vi "Teleop.vi"(10 "Match Info":T1={"Autonomous Elapsed Seconds"=0.0, "TeleOp Elapsed Seconds"=0.0, "Disabled Elapsed Seconds"=0.0, "Visited Autonomous"=FALSE, "Visited TeleOp"=FALSE, "Visited Disabled"=FALSE, "Autonomous Settings"={"Autonomous Style"=enum."Independent", "VI Refnum"=refnum}}, 11 "Call Context":T2=enum."Stop") -> ()   [LabVIEW 2019]
doc: "This VI is called for each enabled TeleOp packet received from the DS. It is typically used to read from joysticks and other inputs and update I/O or setpoints for timed control loops. It should complete and return within 20 milliseconds or risk missing DS packets."
uses:
  <vilib>/Rock Robotics/WPI/DriverStation/WPI_DriverStationDerivedRobotMode.ctl
  <vilib>/Rock Robotics/WPI/DriverStation/WPI_DriverStationMatch Info.ctl
  Typedef/XBox Axis.ctl
  Typedef/XBox Buttons.ctl
  Typedef/XBox POV.ctl
  <vilib>/Rock Robotics/WPI/Utilities/WPI_GetSetVariantRefNum.vi
  <vilib>/Rock Robotics/Network Tables/NT Write Boolean Array.vi
  <vilib>/Rock Robotics/Network Tables/NT Write Numeric Array.vi
panel:
  in  "Winch Speed":dbl=-0.6
  in  "Climb Up Speed":dbl
  in  "Climb Down Speed":dbl
  in  "Queso Arc Sensitivty":dbl=0.5
  in  "QuickTurn Sensitivty":dbl=0.7
  in  "Throttle Sensitivity":dbl=0.5
  in  "max queso power (1)":dbl=1.0
  in  "Trigger Threshold":dbl=0.5 format="%#_13g"
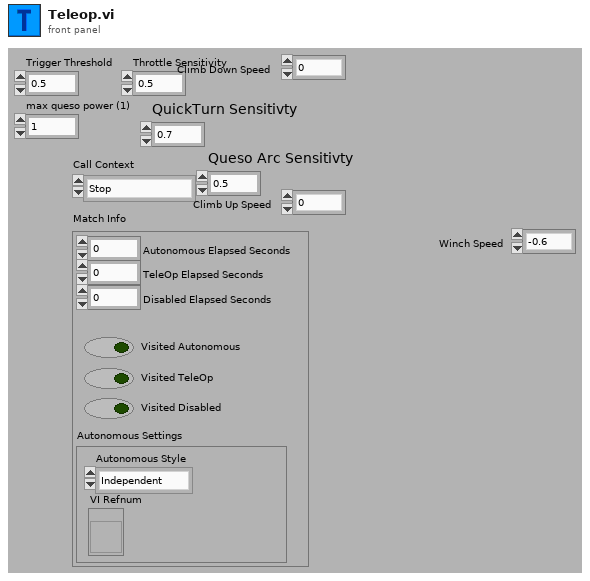
[diagram p1: front panel]
types:
  T1 = typedef "WPI_DriverStationMatch Info.ctl" = cluster{"Autonomous Elapsed Seconds":dbl, "TeleOp Elapsed Seconds":dbl, "Disabled Elapsed Seconds":dbl, "Visited Autonomous":bool, "Visited TeleOp":bool, "Visited Disabled":bool, "Autonomous Settings":cluster{"Autonomous Style":enum16{"Iterative", "Independent"}, "VI Refnum":refnum<vi>}}
  T2 = typedef "WPI_DriverStationDerivedRobotMode.ctl" = enum16{"Init", "Execute", "Stop"}
  T3 = typedef "XBox Buttons.ctl" = enum16{"A", "B", "X", "Y", "Left Bumper", "Right Bumper", "Back", "Start", "Left Joystick", "Right Joystick"}
  T4 = typedef "XBox Axis.ctl" = enum16{"Left X", "Left Y", "Left Trigger", "Right Trigger", "Right X", "Right Y"}
  T5 = typedef "XBox POV.ctl" = enum16{"Center", "Top", "Top Right", "Center Right", "Bottom Right", "Bottom", "Bottom Left", "Center Left", "Top Left"}
  T6 = typedef "WPI_JoystickDevRef.ctl" = cluster{"Device":T7}
  T7 = typedef "WPI_JoystickDeviceEnum.ctl" = enum16{"USB 0", "USB 1", "USB 2", "USB 3", "USB 4", "USB 5"}
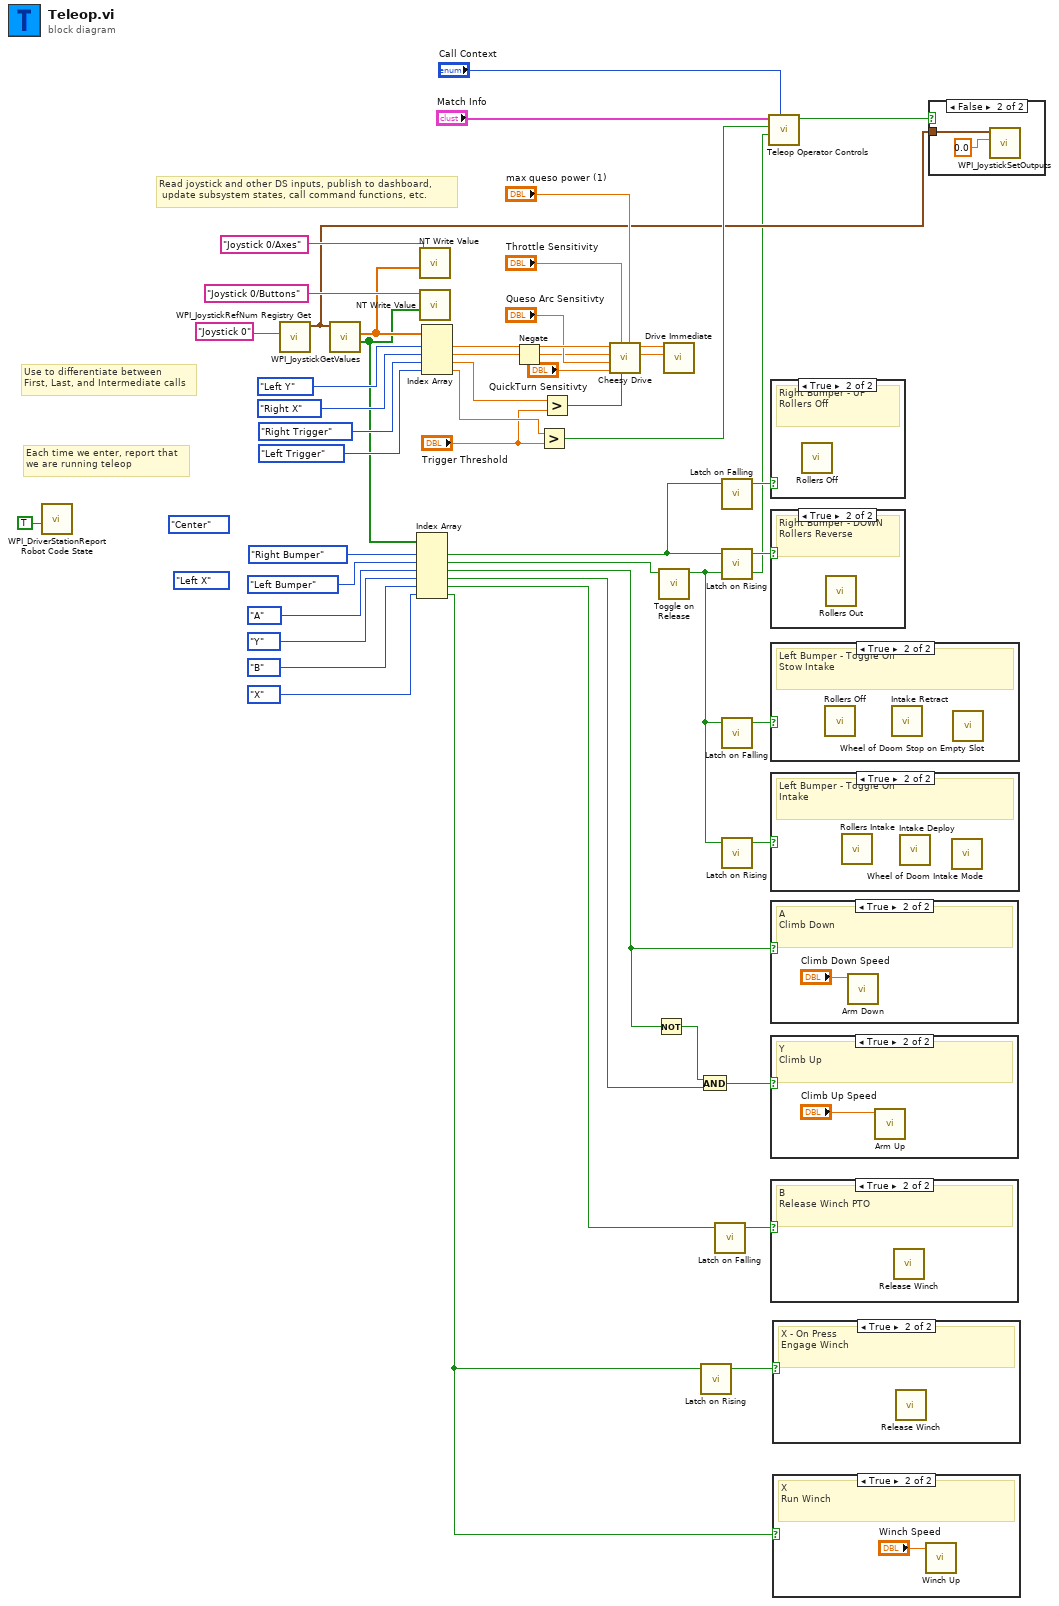
[diagram p0: block diagram]
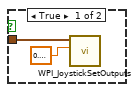
[diagram p7: hidden frame]
diagram:
  (unwired) XBox_Axis."Left X" ("Enum 3")
  (unwired) XBox_POV."Center" ("Enum")
  # "Read joystick and other DS inputs, publish to dashboard,\n update subsystem states, call command functions, etc."
  # "Each time we enter, report that\nwe are running teleop"
  # "Use to differentiate between\nFirst, Last, and Intermediate calls"
  n1 = call <vilib>:"WPI_DriverStationReport Robot Code State.vi"("TeleOp"=TRUE ("Autonomous")) -> ()  [unwired: 10 in, 1 out]
  n2 = call <vilib>:"WPI_JoystickRefNum Registry Get.vi"("refnum name"="Joystick 0") -> ("JoystickDevRef"=w15:T6)  [unwired: 1 in, 9 out]
  n3 = call <vilib>:"WPI_JoystickGetValues.vi"("JoystickDevRef"=w15) -> ("Buttons"=w35:bool[], "Axes"=w46:dbl[])  [unwired: 6 in, 3 out]
  n4 = Index Array(array=w35, index #1=XBox_Buttons."Right Bumper" ("Enum 2"), index #2=XBox_Buttons."Left Bumper" ("Enum 2"), index #3=XBox_Buttons."A" ("Enum 2"), index #4=XBox_Buttons."Y" ("Enum 2"), index #5=XBox_Buttons."B" ("Enum 2"), index #6=XBox_Buttons."X" ("Enum 2")) -> (element #1=w30:bool, element #2=w26:bool, element #3=w8:bool, element #4=w6:bool, element #5=w3:bool, element #6=w1:bool)
  n5 = call-poly <vilib>:"NT Write Value.vi"("Numeric Array"=w46, "Name"="Joystick 0/Axes") -> ()  [unwired: 9 in, 1 out]
  n6 = call-poly <vilib>:"NT Write Value.vi"("Boolean Array"=w35, "Name"="Joystick 0/Buttons") -> ()  [unwired: 9 in, 1 out]
  n7 = Index Array(array=w46, index #1=XBox_Axis."Left Y" ("Enum"), index #2=XBox_Axis."Right X" ("Enum"), index #3=XBox_Axis."Right Trigger" ("Enum"), index #4=XBox_Axis."Left Trigger" ("Enum")) -> (element #1=w39:dbl, element #2=w38:dbl, element #3=w34:dbl, element #4=w25:dbl)
  n8 = Negate(x=w38) -> (-x=w18:dbl)
  n9 = Greater?(x=w25, y="Trigger Threshold") -> (0:w23:bool)
  n10 = Greater?(x=w34, y="Trigger Threshold") -> (0:w33:bool)
  n11 = call <vilib>:"Cheesy Drive.vi"("max queso power (1)"="max queso power (1)", "Quickturn"=w33, "Throttle Sensitivity"="Throttle Sensitivity", "QuickTurn Sensitivty"="QuickTurn Sensitivty", "Queso Arc Sensitivty"="Queso Arc Sensitivty", "Wheel"=w18, "Throttle"=w39) -> ("Right PWM"=w36:dbl, "Left PWM"=w37:dbl)  [unwired: 3 in]
  n12 = Not(x=w8) -> (.not. x?=w7:bool)
  n13 = call <vilib>:"Toggle on Release.vi"("Boolean"=w26) -> ("toggle on release"=w14:bool)  [unwired: 10 in]
  n14 = call "Drive Immediate.vi"("Right Setpoint"=w36, "Left Setpoint"=w37) -> ()  [unwired: 9 in, 1 out]
  n15 = And(x=w7, y=w6) -> (x .and. y?=w5:bool)
  n16 = call <vilib>:"Latch on Rising.vi"("Boolean in"=w1) -> ("Boolean out"=w2:bool)  [unwired: 4 in]
  n17 = call <vilib>:"Latch on Falling.vi"("Boolean in"=w3) -> ("Boolean out"=w4:bool)  [unwired: 4 in]
  n18 = call <vilib>:"Latch on Falling.vi"("Boolean in"=w30) -> ("Boolean out"=w31:bool)  [unwired: 4 in]
  n19 = call <vilib>:"Latch on Rising.vi"("Boolean in"=w30) -> ("Boolean out"=w29:bool)  [unwired: 4 in]
  n20 = call <vilib>:"Latch on Falling.vi"("Boolean in"=w14) -> ("Boolean out"=w27:bool)  [unwired: 4 in]
  n21 = call <vilib>:"Latch on Rising.vi"("Boolean in"=w14) -> ("Boolean out"=w28:bool)  [unwired: 4 in]
  n22 = call "Teleop Operator Controls.vi"("Call Context"="Call Context", "Intaking"=w14, "Driver Agree To Shoot? (F)"=w23, "Match Info"="Match Info") -> ("Operator Ready To Shoot?"=w16:bool)  [unwired: 7 in]
  n23 = case shown="True" w31 {
    frame False {
    }
    frame True {
      # "Right Bumper - UP\nRollers Off"
      n24 = call "Rollers Off.vi"() -> ()  [unwired: 11 in, 1 out]
    }
  }
  n25 = case shown="True" w29 {
    frame False {
    }
    frame True {
      # "Right Bumper - DOWN\nRollers Reverse"
      n26 = call "Rollers Out.vi"() -> ()  [unwired: 11 in, 1 out]
    }
  }
  n27 = case shown="True" w27 {
    frame False {
    }
    frame True {
      # "Left Bumper - Toggle Off\nStow Intake"
      n28 = call "Rollers Off.vi"() -> ()  [unwired: 11 in, 1 out]
      n29 = call "Intake Retract.vi"() -> ()  [unwired: 11 in, 1 out]
      n30 = call "Wheel of Doom Stop on Empty Slot.vi"() -> ()  [unwired: 11 in, 1 out]
    }
  }
  n31 = case shown="True" w28 {
    frame False {
    }
    frame True {
      # "Left Bumper - Toggle On\nIntake"
      n32 = call "Rollers Intake.vi"() -> ()  [unwired: 11 in, 1 out]
      n33 = call "Intake Deploy.vi"() -> ()  [unwired: 11 in, 1 out]
      n34 = call "Wheel of Doom Intake Mode.vi"() -> ()  [unwired: 11 in, 1 out]
    }
  }
  n35 = case shown="True" w8 {
    frame False {
    }
    frame True {
      # "A\nClimb Down"
      n36 = call "Arm Down.vi"("Setpoint"="Climb Down Speed") -> ()  [unwired: 10 in, 1 out]
    }
  }
  n37 = case shown="True" w5 {
    frame False {
    }
    frame True {
      # "Y\nClimb Up"
      n38 = call "Arm Up.vi"("Setpoint"="Climb Up Speed") -> ()  [unwired: 10 in, 1 out]
    }
  }
  n39 = case shown="True" w4 {
    frame False {
    }
    frame True {
      # "B\nRelease Winch PTO"
      n40 = call "Release Winch.vi"() -> ()  [unwired: 11 in, 1 out]
    }
  }
  n41 = case shown="True" w2 {
    frame False {
    }
    frame True {
      # "X - On Press\nEngage Winch"
      n42 = call "Release Winch.vi"() -> ()  [unwired: 11 in, 1 out]
    }
  }
  n43 = case shown="True" w1 {
    frame False {
    }
    frame True {
      # "X\nRun Winch"
      n44 = call "Winch Up.vi"("Setpoint"="Winch Speed") -> ()  [unwired: 10 in, 1 out]
    }
  }
  n45 = case shown="False" w16 {
    tunnel: w15 -> [w54 w56]
    frame True {
      n46 = call <vilib>:"WPI_JoystickSetOutputs.vi"("Left Rumble"=sgl 0.3, "JoystickDevRef"=w54) -> ()  [unwired: 8 in, 2 out]
    }
    frame False {
      n47 = call <vilib>:"WPI_JoystickSetOutputs.vi"("Left Rumble"=sgl 0.0, "JoystickDevRef"=w56) -> ()  [unwired: 8 in, 2 out]
    }
  }
